vi "1 Channel 1 Sample - Manual Timestamps.vi"() -> ()   [LabVIEW 2026, in "synnax_clib.lvlib"]
uses:
  synnax_clib.lvlib
  typedefs/connection_config.ctl
  classes/Writer/Private/Writes/DBL/Write 1Ch 1Samp (DBL).vi
  classes/Writer/Private/synnax writer open Array.vi
  classes/Client/Private/synnax channel retrieve keys Array.vi
  classes/Synnax Writer.lvclass
  classes/Client/Synnax Client.lvclass
panel:
  in  "Channels":string[](array[numeric])=["my_f64_chan", "my_f64_idx"]
  out "cos(x)":dbl
  in  "Stop":bool
  out "error out":errorcluster
  in  "Connection Config":T1={"host"="localhost", "port"=9090, "username"="synnax", "password"="seldon"}
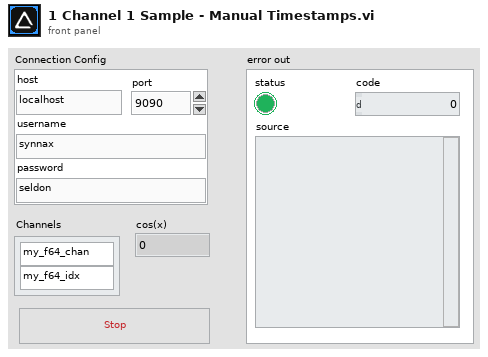
[diagram p1: front panel]
types:
  T1 = typedef "synnax_clib.lvlib/connection_config.ctl" = cluster{"host":string, "port":u16, "username":string, "password":string}
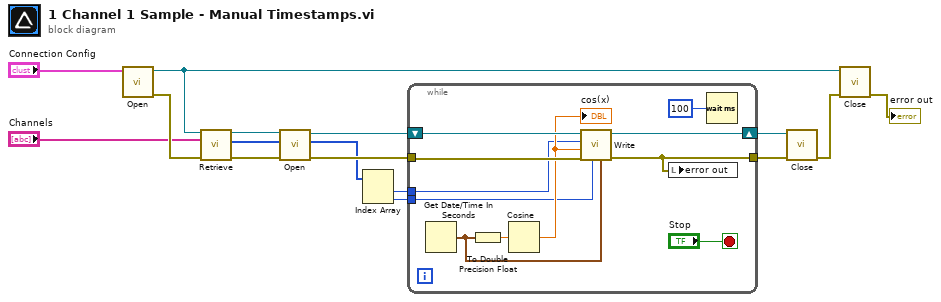
[diagram p0: block diagram]
diagram:
  n1 = call "Open.vi"("Connection Config"="Connection Config") -> ("error out"=w11:errorcluster, "Synnax Client out"=w13:refnum<class "Synnax Client.lvclass">)  [unwired: 9 in]
  n2 = call-poly "Retrieve.vi"("Synnax Client in"=w13, "channel names"="Channels", "error in"=w11) -> ("Synnax Client out"=w7:refnum<class "Synnax Client.lvclass">, "channel keys"=w6:u32[], "error out"=w15:errorcluster)  [unwired: 9 in, 1 out]
  n3 = call-poly "Open.vi"("error in"=w15, "channels in"=w6, "Synnax Client in"=w7) -> ("error out"=w8:errorcluster, "channels out"=w3:u32[], "writer out"=w10:refnum<class "Synnax Writer.lvclass">)  [unwired: 6 in]
  n4 = Index Array(array=w3) -> (element #1=w2:u32, element #2=w1:u32)  [unwired: 2 in]
  n5 = while {
    shift-right: [w26] -> w9
    shift-left: w10 -> [w27]
    tunnel: w8 -> [w25]
    tunnel: [w21] -> w16
    tunnel: w2 -> [w19]
    tunnel: w1 -> [w18]
    stop <- "Stop" stop-if-true
    n6 = Get Date/Time In Seconds() -> (seconds since 1Jan1904=w17:timestamp)
    n7 = To Double Precision Float(number=w17) -> (double precision float=w20:dbl)
    n8 = Cosine(x=w20) -> (cos(x)=w23:dbl)
    "cos(x)" <- w23
    n9 = call-poly "Write.vi"("timestamp"=w17, "index_channel"=w18, "error in"=w25, "data"=w23, "channel"=w19, "Writer"=w27) -> ("error out"=w21:errorcluster, "Writer Out"=w26:refnum<class "Synnax Writer.lvclass">)  [unwired: 4 in]
    n10 = local write "error out"(w21) -> ()
    n11 = Wait (ms)(milliseconds to wait=u32 100) -> ()  [unwired: 1 out]
  }
  n12 = call "Close.vi"("error in"=w16, "writer"=w9) -> ("error out"=w12:errorcluster)  [unwired: 9 in]
  n13 = call "Close.vi"("error in"=w12, "Synnax Client in"=w13) -> ("error out"=→"error out":errorcluster)  [unwired: 9 in]
